vi "Set Frequency Parameters.vi"(8 "error in (no error)":errorcluster, 10 "Step In":refnum<k7>, 11 "Skyworks Spur Test in":refnum<class "Skyworks Spur Test.lvclass">) -> (0 "error out":errorcluster, 2 "Step Out":refnum<k7>, 3 "Skyworks Spur Test out":refnum<class "Skyworks Spur Test.lvclass">)   [LabVIEW 2018, in "Skyworks Spur Test.lvlib" / "Skyworks Spur Test.lvclass"]
uses:
  Skyworks Spur Test.lvclass
  Skyworks Spur Test.lvclass/Skyworks Spur Test.ctl
  Read SG Parameters.vi
  Read SA Parameters.vi
  Plugins/TestStand API Tools (TSAT).lvlibp/Step Actions/TSAT Step Actions.lvlib
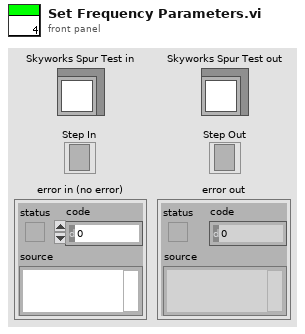
[diagram p1: front panel]
types:
  T1 = cluster{"Start Frequency":dbl, "Stop Frequency":dbl, "Delta":dbl}
  T2 = typedef "Skyworks Spur Test.lvlib/Skyworks Spur Test.lvclass/SA Parameters.ctl" = cluster{"Start Frequency":dbl, "Stop Frequency":dbl, "Bandwidth":dbl}
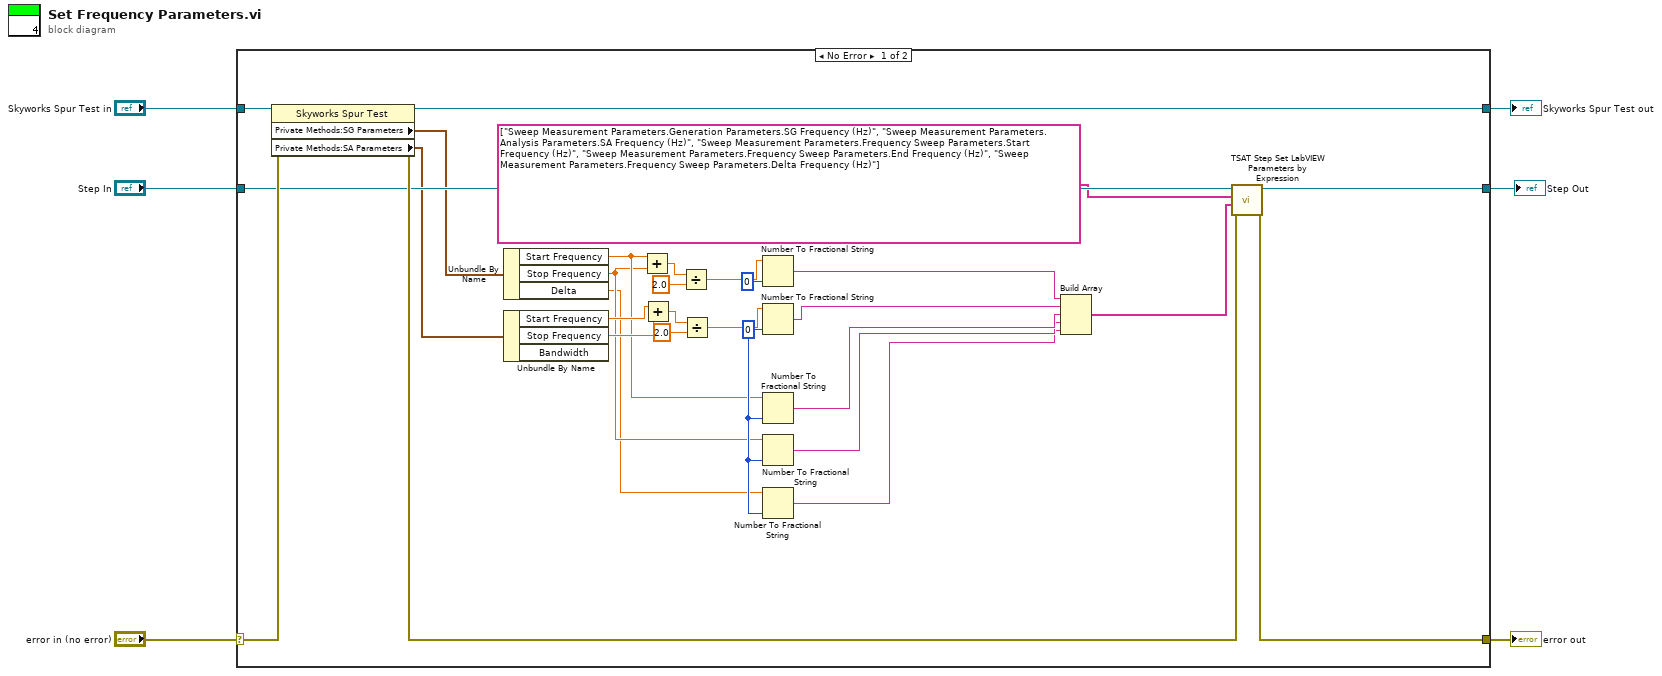
[diagram p0: block diagram]
diagram:
  n1 = case shown="No Error" "error in (no error)" {
    selector: "error in (no error)" -> [w35 w38]
    tunnel: [w31 w38] -> w5
    tunnel: [w33 w37] -> w3
    tunnel: "Skyworks Spur Test in" -> [w34 w37]
    tunnel: "Step In" -> [w30 w36]
    tunnel: [w29 w36] -> w1
    frame No Error {
      w15 = i16 0 ("precision (6)")
      n2 = property class="Skyworks Spur Test"(reference=w34, error in=w35) -> (reference out=w33:refnum<class "Skyworks Spur Test.lvclass">, error out=w32:errorcluster, "Private Methods:SG Parameters"=w26:T1, "Private Methods:SA Parameters"=w25:T2)
      n3 = Unbundle By Name(w26) -> ("Start Frequency"=w12:dbl, "Stop Frequency"=w11:dbl, "Delta"=w10:dbl)
      n4 = Unbundle By Name(w25) -> ("Start Frequency"=w14:dbl, "Stop Frequency"=w13:dbl)  [unwired: 1 out]
      n5 = Add(x=w12, y=w11) -> (x+y=w17:dbl)
      n6 = Add(x=w14, y=w13) -> (x+y=w24:dbl)
      n7 = Divide(x=w17, y=2.0) -> (x/y=w19:dbl)
      n8 = Divide(x=w24, y=2.0) -> (x/y=w22:dbl)
      n9 = Number To Fractional String(number=w19, precision (6)=i16 0) -> (F-format string=w16:string)  [unwired: 2 in]
      n10 = Number To Fractional String(number=w22, precision (6)=w15) -> (F-format string=w21:string)  [unwired: 2 in]
      n11 = Number To Fractional String(number=w12, precision (6)=w15) -> (F-format string=w9:string)  [unwired: 2 in]
      n12 = Number To Fractional String(number=w11, precision (6)=w15) -> (F-format string=w8:string)  [unwired: 2 in]
      n13 = Number To Fractional String(number=w10, precision (6)=w15) -> (F-format string=w7:string)  [unwired: 2 in]
      n14 = Build Array(w16, w21, w9, w8, w7) -> (w27:string[])
      n15 = call "TSAT Step Set LabVIEW Parameters by Expression.vi"("Error In"=w32, "Value Expressions"=w27, "Parameters to Set"=string[] ["Sweep Measurement Parameters.Generation Parameters.SG Frequency (Hz)", "Sweep Measurement Parameters.Analysis Parameters.SA Frequency (Hz)", "Sweep Measurement Parameters.Frequency Sweep Parameters.Start Frequency (Hz)", "Sweep Measurement Parameters.Frequency Sweep Parameters.End Frequency (Hz)", "Sweep Measurement Parameters.Frequency Sweep Parameters.Delta Frequency (Hz)"], "Step In"=w30) -> ("Error Out"=w31:errorcluster, "Step Out"=w29:refnum<k7>)  [unwired: 6 in]
    }
    frame Error {
    }
  }
  "error out" <- w5
  "Skyworks Spur Test out" <- w3
  "Step Out" <- w1
